vi "FL Get Variable.vi"(0 "fuzzy system in":T4 {"user MF interpolating polynomials"."coa_x(y) coeff" format="%.4g"; "user MF interpolating polynomials"."Area(y) coeff" format="%.4g"; "user MF interpolating polynomials"."X(y) coeff" format="%.4g"; "user MF interpolating polynomials"."Y(x) coeff" format="%.4g"; "user MF interpolating polynomials"."Y" format="%.4g"; "user MF interpolating polynomials"."X" format="%.4g"; "defuzzification method" items=["Center of Area", "Modified Center of Area", "Center of Sums", "Center of Maximum", "Mean of Maximum"]; "rules"."consequents"."Var Index" min=0; "rules"."consequents"."Cond" items=["=", "!="]; "rules"."consequents"."MF Index" min=0; "rules"."antecedents"."Var Index" min=0; "rules"."antecedents"."Cond" items=["=", "!="]; "rules"."antecedents"."MF Index" min=0; "rules"."consequent implication" items=["Minimum", "Product"]; "rules"."antecedent connective" items=["AND (Minimum)", "AND (Product)", "OR (Maximum)", "OR (Probabilistic)"]; "output variables"."MFs"."shape" items=["Triangle", "Trapezoid", "Singleton", "Sigmoid", "Gaussian", "User-Defined"]; "input variables"."MFs"."shape" items=["Triangle", "Trapezoid", "Singleton", "Sigmoid", "Gaussian", "User-Defined"]}, 1 "input/output":T1 items=["Input", "Output"], 2 "variable index":i32, 11 "error in (no error)":errorcluster) -> (4 "fuzzy system out":T4 {"user MF interpolating polynomials"."coa_x(y) coeff" format="%.4g"; "user MF interpolating polynomials"."Area(y) coeff" format="%.4g"; "user MF interpolating polynomials"."X(y) coeff" format="%.4g"; "user MF interpolating polynomials"."Y(x) coeff" format="%.4g"; "user MF interpolating polynomials"."Y" format="%.4g"; "user MF interpolating polynomials"."X" format="%.4g"; "defuzzification method" items=["Center of Area", "Modified Center of Area", "Center of Sums", "Center of Maximum", "Mean of Maximum"]; "rules"."consequents"."Var Index" min=0; "rules"."consequents"."Cond" items=["=", "!="]; "rules"."consequents"."MF Index" min=0; "rules"."antecedents"."Var Index" min=0; "rules"."antecedents"."Cond" items=["=", "!="]; "rules"."antecedents"."MF Index" min=0; "rules"."consequent implication" items=["Minimum", "Product"]; "rules"."antecedent connective" items=["AND (Minimum)", "AND (Product)", "OR (Maximum)", "OR (Probabilistic)"]; "output variables"."MFs"."shape" items=["Triangle", "Trapezoid", "Singleton", "Sigmoid", "Gaussian", "User-Defined"]; "input variables"."MFs"."shape" items=["Triangle", "Trapezoid", "Singleton", "Sigmoid", "Gaussian", "User-Defined"]}, 6 "name":string, 8 "minimum":dbl, 10 "maximum":dbl, 14 "membership functions":T2[](array[typedef]) {"shape" items=["Triangle", "Trapezoid", "Singleton", "Sigmoid", "Gaussian", "User-Defined"]}, 15 "error out":errorcluster)   [LabVIEW 2017, in "NI_Fuzzy_Logic_API.lvlib"]
doc: "Returns the name, range, and membership functions for a linguistic variable in a fuzzy system."
uses:
  <vilib>/addons/Fuzzy Logic/NI_Fuzzy_Logic_API.lvlib
  <vilib>/addons/Fuzzy Logic/TypeDefs/FL System.ctl
  <vilib>/addons/Fuzzy Logic/TypeDefs/FL Variable.ctl
  <vilib>/addons/Fuzzy Logic/TypeDefs/FL Membership Function.ctl
  <vilib>/addons/Fuzzy Logic/TypeDefs/FL Membership Function Shape.ctl
  <vilib>/addons/Fuzzy Logic/TypeDefs/FL Rule.ctl
  <vilib>/addons/Fuzzy Logic/TypeDefs/FL Antecedent.ctl
  <vilib>/addons/Fuzzy Logic/TypeDefs/FL Modifier.ctl
  <vilib>/addons/Fuzzy Logic/TypeDefs/FL Antecedent Connective.ctl
  <vilib>/addons/Fuzzy Logic/TypeDefs/FL Consequent.ctl
  <vilib>/addons/Fuzzy Logic/TypeDefs/FL Consequent Implication.ctl
  <vilib>/addons/Fuzzy Logic/TypeDefs/FL Defuzzification.ctl
  <vilib>/addons/Fuzzy Logic/TypeDefs/FL Interpolating polynomials.ctl
  <vilib>/addons/Fuzzy Logic/TypeDefs/FL Input_Output.ctl
panel:
  # "IF"
  # "THEN"
  # "IF"
  # "THEN"
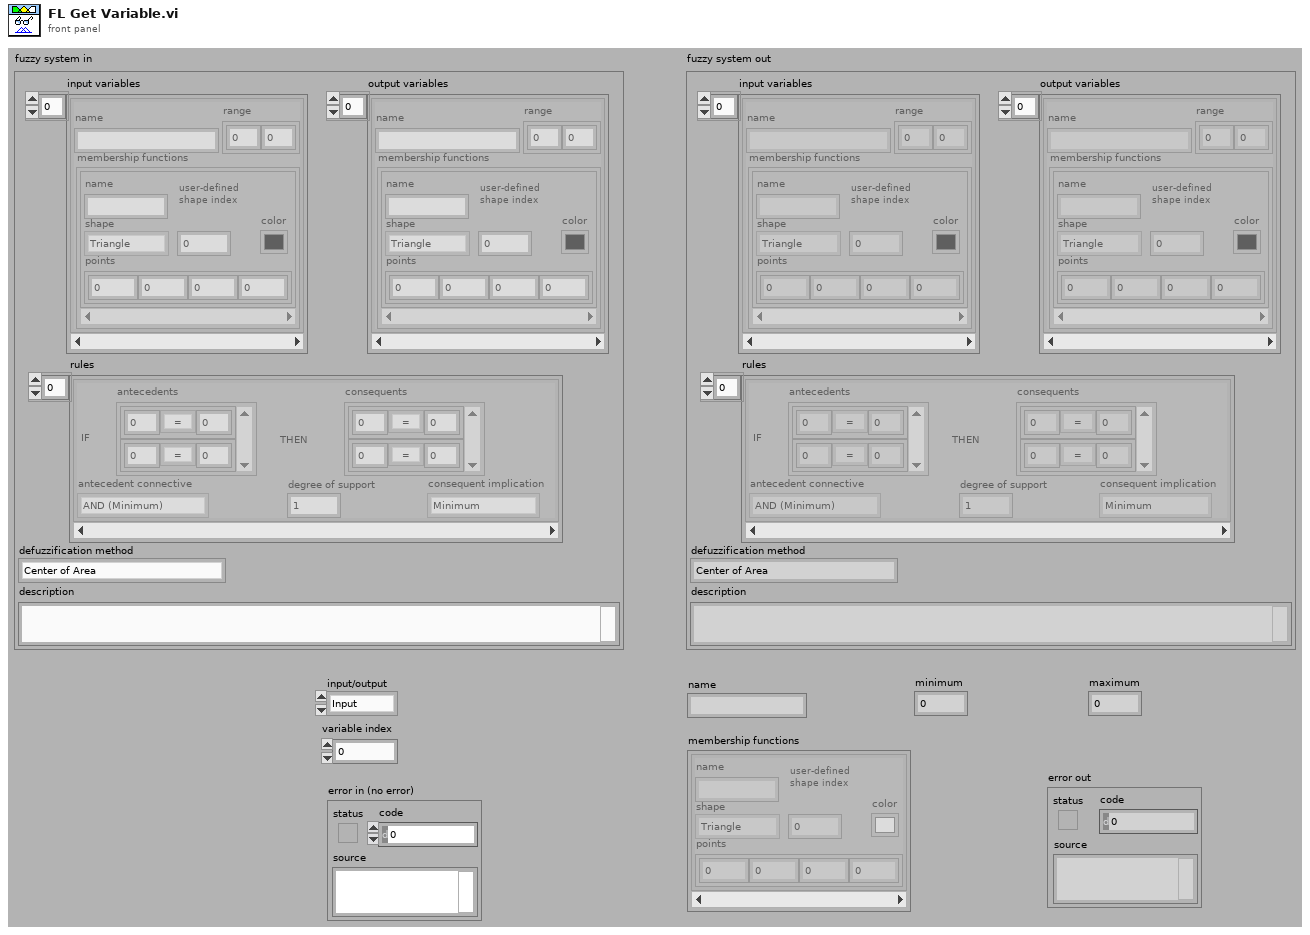
[diagram p1: front panel]
types:
  T1 = typedef "NI_Fuzzy_Logic_API.lvlib/FL Input_Output.ctl" = u16
  T2 = typedef "NI_Fuzzy_Logic_API.lvlib/FL Membership Function.ctl" = cluster{"name":string, "shape":T3, "points":dbl[], "color":u32, "user-defined shape index":i32}
  T3 = typedef "NI_Fuzzy_Logic_API.lvlib/FL Membership Function Shape.ctl" = u16
  T4 = typedef "NI_Fuzzy_Logic_API.lvlib/FL System.ctl" = cluster{"input variables":T5[], "output variables":T5[], "rules":T6[], "defuzzification method":T12, "description":string, "user MF interpolating polynomials":T13[]}
  T5 = typedef "NI_Fuzzy_Logic_API.lvlib/FL Variable.ctl" = cluster{"name":string, "range":dbl[], "MFs":T2[]}
  T6 = typedef "NI_Fuzzy_Logic_API.lvlib/FL Rule.ctl" = cluster{"antecedents":T7[], "antecedent connective":T9, "consequents":T10[], "consequent implication":T11, "degree of support":dbl}
  T7 = typedef "NI_Fuzzy_Logic_API.lvlib/FL Antecedent.ctl" = cluster{"Var Index":i32, "MF Index":i32, "Cond":T8}
  T8 = typedef "NI_Fuzzy_Logic_API.lvlib/FL Modifier.ctl" = u16
  T9 = typedef "NI_Fuzzy_Logic_API.lvlib/FL Antecedent Connective.ctl" = u16
  T10 = typedef "NI_Fuzzy_Logic_API.lvlib/FL Consequent.ctl" = cluster{"Var Index":i32, "MF Index":i32, "Cond":T8}
  T11 = typedef "NI_Fuzzy_Logic_API.lvlib/FL Consequent Implication.ctl" = u16
  T12 = typedef "NI_Fuzzy_Logic_API.lvlib/FL Defuzzification.ctl" = u16
  T13 = typedef "NI_Fuzzy_Logic_API.lvlib/FL Interpolating polynomials.ctl" = cluster{"X":dbl[], "Y":dbl[], "Y(x) coeff":dbl[][], "X(y) coeff":dbl[][], "Area(y) coeff":dbl[][], "coa_x(y) coeff":dbl[][]}
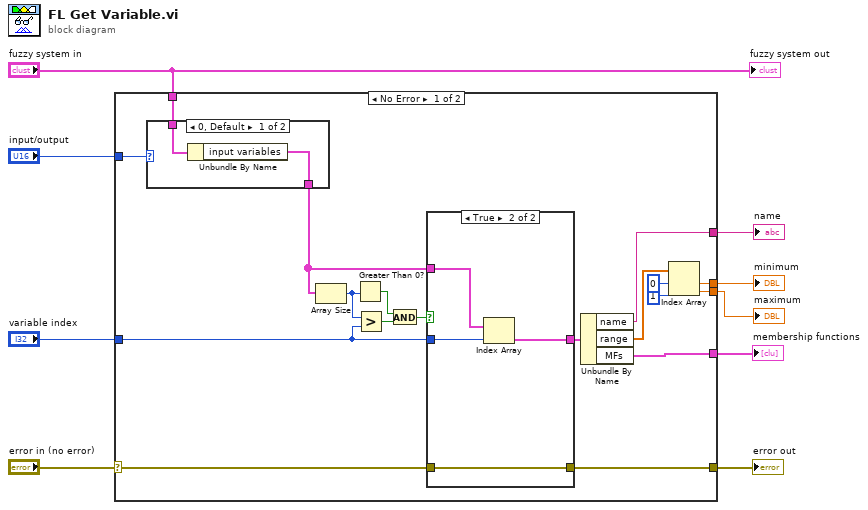
[diagram p0: block diagram]
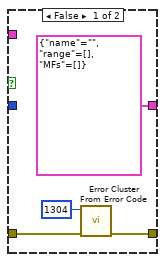
[diagram p2: hidden frame]
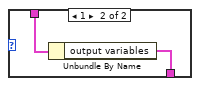
[diagram p3: hidden frame]
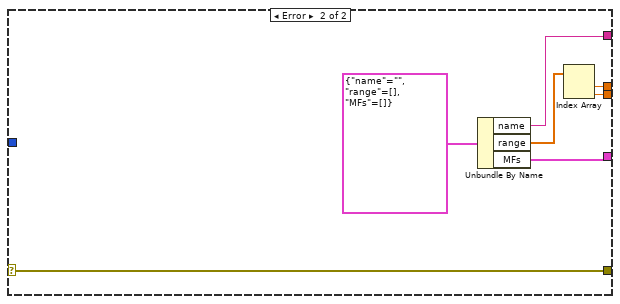
[diagram p4: hidden frame]
diagram:
  n1 = case shown="No Error" "error in (no error)" {
    selector: "error in (no error)" -> [w16 w46]
    tunnel: "fuzzy system in" -> [w27 _]
    tunnel: "variable index" -> [w18 _]
    tunnel: [w25 w44] -> w6
    tunnel: [w24 w43] -> w7
    tunnel: "input/output" -> [w23 _]
    tunnel: [w17 w46] -> w8
    tunnel: [w11 w41] -> w2
    tunnel: [w10 w40] -> w1
    frame No Error {
      n2 = case shown="0, Default" w23 {
        tunnel: w27 -> [w37 w39]
        tunnel: [w36 w38] -> w19
        frame 0, Default {
          n3 = Unbundle By Name(w37) -> ("input variables"=w36:T5[])
        }
        frame 1 {
          n4 = Unbundle By Name(w39) -> ("output variables"=w38:T5[])
        }
      }
      n5 = Array Size(array=w19) -> (size(s)=w21:i32)
      n6 = Greater Than 0?(x=w21) -> (x > 0?=w20:bool)
      n7 = Greater?(x=w21, y=w18) -> (0:w22:bool)
      n8 = And(x=w20, y=w22) -> (x .and. y?=w15:bool)
      n9 = case shown="True" w15 {
        tunnel: [T5 {"name"="", "range"=[], "MFs"=[]} ("Variable") w35] -> w26
        tunnel: w19 -> [_ w34]
        tunnel: w18 -> [_ w33]
        tunnel: [w29 w32] -> w17
        tunnel: w16 -> [w30 w32]
        frame False {
          n10 = call <vilib>:"Error Cluster From Error Code.vi"("error in (no error)"=w30, "error code (0)"=1304) -> ("error out"=w29:errorcluster)  [unwired: 1 in, 6 out]
        }
        frame True {
          n11 = Index Array(array=w34, index=w33) -> (element=w35:T5)
        }
      }
      n12 = Unbundle By Name(w26) -> ("name"=w25:string, "range"=w14:dbl[], "MFs"=w24:T2[])
      n13 = Index Array(array=w14, index #1=0 ("index"), index #2=1 ("index")) -> (element #1=w11:dbl, element #2=w10:dbl)
    }
    frame Error {
      n14 = Unbundle By Name(T5 {"name"="", "range"=[], "MFs"=[]} ("Variable")) -> ("name"=w44:string, "range"=w42:dbl[], "MFs"=w43:T2[])
      n15 = Index Array(array=w42) -> (element #1=w41:dbl, element #2=w40:dbl)  [unwired: 2 in]
    }
  }
  "name" <- w6
  "membership functions" <- w7
  "error out" <- w8
  "maximum" <- w1
  "minimum" <- w2
  "fuzzy system out" <- "fuzzy system in"
